vi "PromptUserFileExists.vi"(0 "Project":string, 1 "Measurement Description":string, 2 "Measurement Number":i32) -> (3 "Project":string, 4 "Measurement Description":string, 5 "Measurement Number":i32, 6 "Overwrite":bool)   [LabVIEW 2018]
doc: "Displays a standard dialog box that prompts users to enter information, such as a user name and password.\n--------------------\n\nThis Express VI is configured as follows:\n\nMessage to Display to the User:\nThe inputs are: \nText Entry Box: Project\nText Entry Box: Measurement Description\nNumber: Measurement Number"
panel:
  out "error out":errorcluster
  in  "error in (no error)":errorcluster
  out "String":string
  in  "Enable":bool=TRUE
  in  "Cancel":bool
  in  "OK2":bool
  in  "OK1":bool
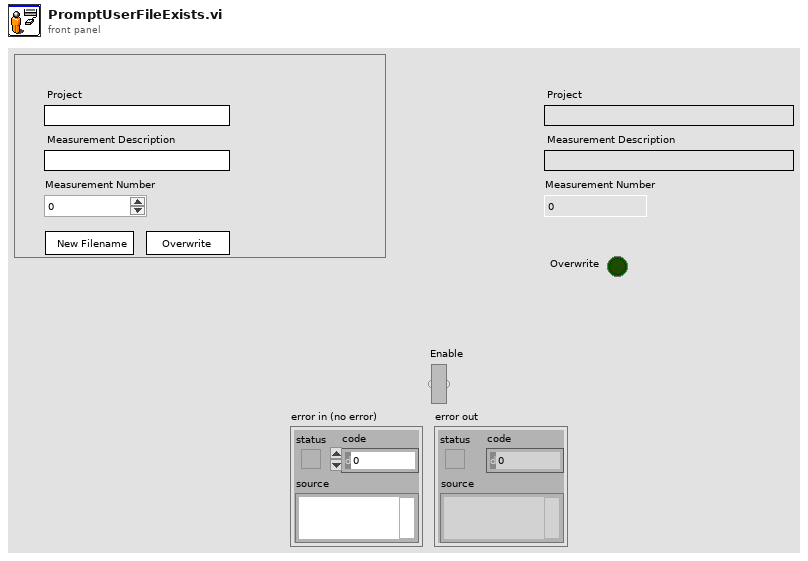
[diagram p1: front panel]
types:
  T1 = cluster{"Input Name":string, "Input Data Type":i32}[]
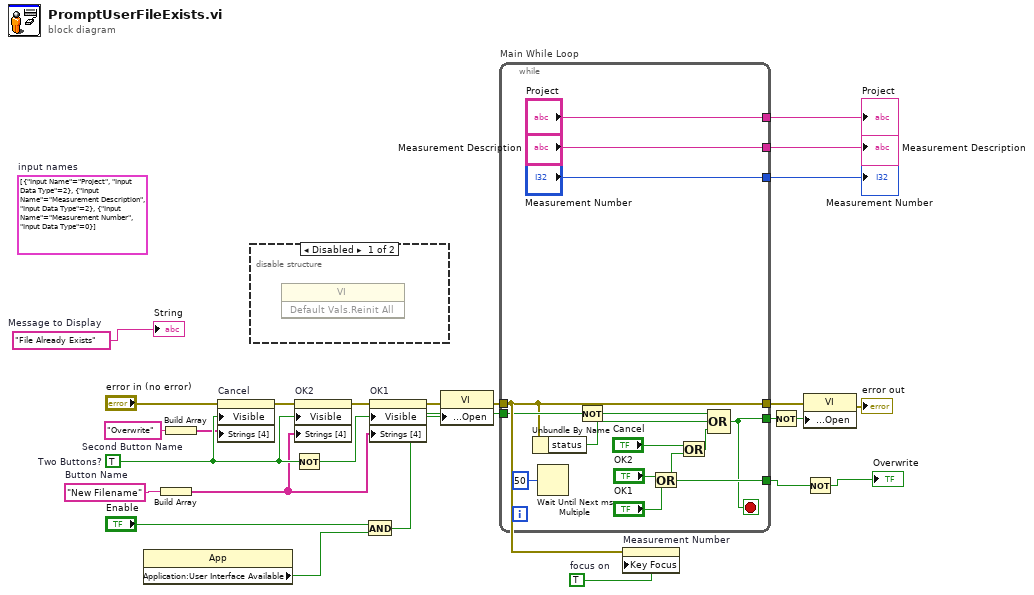
[diagram p0: block diagram]
diagram:
  w6 = TRUE  # focus on
  (unwired) T1 [{"Input Name"="Project", "Input Data Type"=2}, {"Input Name"="Measurement Description", "Input Data Type"=2}, {"Input Name"="Measurement Number", "Input Data Type"=0}]  # input names
  w18 = "Overwrite"  # Second Button Name
  w16 = "New Filename"  # Button Name
  w3 = "File Already Exists"  # Message to Display
  w25 = TRUE  # Two Buttons?
  n1 = property class="App"() -> ("Application:User Interface Available"=w8:bool)  [unwired: 2 in, 2 out]
  n2 = Build Array(w16) -> (w17:string[])
  n3 = Build Array(w18) -> (w19:string[])
  n4 = property on="Cancel" class="Bool"(error in="error in (no error)", "Visible"=w25, "Strings [4]"=w19) -> (error out=w23:errorcluster)  [unwired: 1 in, 1 out]
  n5 = disable-structure shown="Disabled" {
    frame Disabled {
      n6 = invoke class="VI" method="Default Vals.Reinit All"() -> ()  [unwired: 3 in, 3 out]
    }
    frame Enabled {
    }
  }
  n7 = Not(x=w25) -> (.not. x?=w24:bool)
  n8 = property on="OK2" class="Bool"(error in=w23, "Visible"=w25, "Strings [4]"=w17) -> (error out=w22:errorcluster)  [unwired: 1 in, 1 out]
  n9 = And(x="Enable", y=w8) -> (x .and. y?=w9:bool)
  n10 = property on="OK1" class="Bool"(error in=w22, "Visible"=w24, "Strings [4]"=w17) -> (error out=w15:errorcluster)  [unwired: 1 in, 1 out]
  n11 = property class="VI"(error in=w15, "Front Panel Window:Open"=w9) -> (error out=w14:errorcluster)  [unwired: 1 in, 1 out]
  n12 = while "Main While Loop" {
    tunnel: [w36] -> w2
    tunnel: w9 -> [w34]
    tunnel: [w32] -> w20
    tunnel: w14 -> [w31]
    tunnel: [w31] -> w12
    tunnel: ["Project"] -> w7
    tunnel: ["Measurement Description"] -> w5
    tunnel: ["Measurement Number"] -> w4
    stop <- w32 stop-if-true
    n13 = Unbundle By Name(w31) -> ("status"=w29:bool)
    n14 = Wait Until Next ms Multiple(millisecond multiple=u32 50) -> ()  [unwired: 1 out]
    n15 = Not(x=w34) -> (.not. x?=w33:bool)
    n16 = Or(x="OK2", y="OK1") -> (x .or. y?=w36:bool)
    n17 = Or(x="Cancel", y=w36) -> (x .or. y?=w30:bool)
    n18 = Compound Arithmetic op=OR(w33, w29, w30) -> (w32:bool)
  }
  "Project" <- w7
  "Measurement Description" <- w5
  "Measurement Number" <- w4
  n19 = property on="Measurement Number" class="DigNum (strict)"(error in=w14, "Key Focus"=w6) -> ()  [unwired: 1 in, 2 out]
  n20 = Not(x=w20) -> (.not. x?=w21:bool)
  n21 = property class="VI"(error in=w12, "Front Panel Window:Open"=w21) -> (error out=→"error out":errorcluster)  [unwired: 1 in, 1 out]
  n22 = Not(x=w2) -> (.not. x?=→"Overwrite":bool)
  "String" <- w3
